vi "Add Data to Table.vi"(10 "User Data":T1(array[cluster])=[{"User ID (key)"=0, "First Name"="Dude", "Last Name"="marlow", "Extension"="", "Department"="", "Citizenship"="", "Company"="", "GDLS Employee"=FALSE, "Foreign National"=FALSE}, {"User ID (key)"=0, "First Name"="Where's", "Last Name"="Nowak", "Extension"="", "Department"="", "Citizenship"="", "Company"="", "GDLS Employee"=FALSE, "Foreign National"=FALSE}, {"User ID (key)"=0, "First Name"="My", "Last Name"="Jones", "Extension"="", "Department"="", "Citizenship"="", "Company"="", "GDLS Employee"=FALSE, "Foreign National"=FALSE}, {"User ID (key)"=0, "First Name"="Car", "Last Name"="Hofer", "Extension"="", "Department"="", "Citizenship"="", "Company"="", "GDLS Employee"=FALSE, "Foreign National"=FALSE}, {"User ID (key)"=0, "First Name"="Man", "Last Name"="Murphy", "Extension"="", "Department"="", "Citizenship"="", "Company"="", "GDLS Employee"=FALSE, "Foreign National"=FALSE}]) -> ()   [LabVIEW 2011]
uses:
  System.Windows.Forms
  System.Data
panel:
  out "CurrentRowIndex":i32
  in  "stop":bool
  in  ".NET Container":refnum<k24>(container)
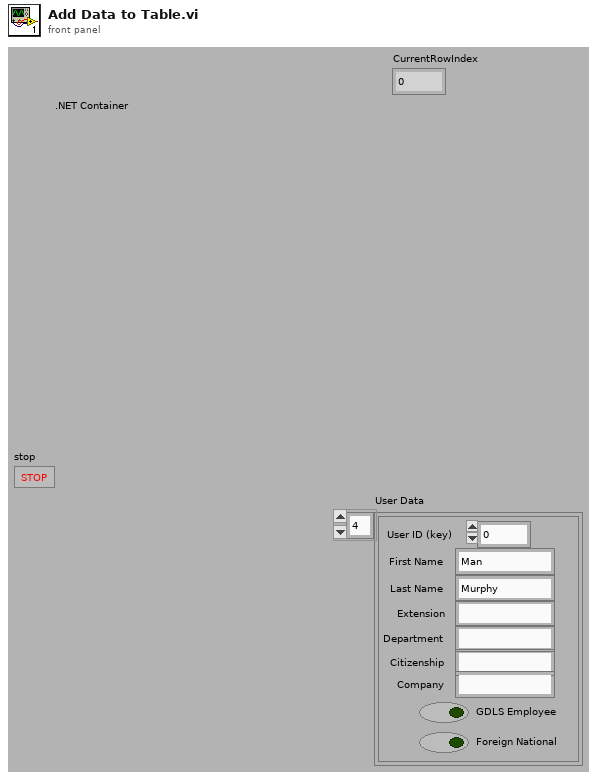
[diagram p1: front panel]
types:
  T1 = cluster{"User ID (key)":i32, "First Name":string, "Last Name":string, "Extension":string, "Department":string, "Citizenship":string, "Company":string, "GDLS Employee":bool, "Foreign National":bool}[]
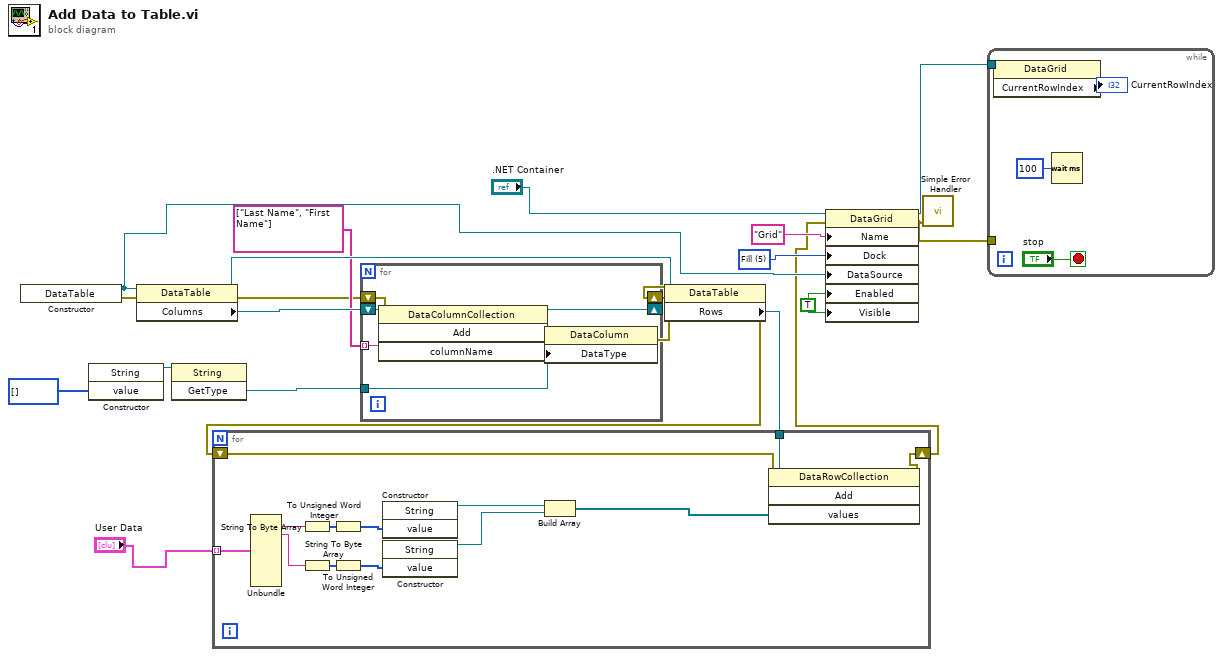
[diagram p0: block diagram]
diagram:
  w9 = TRUE ("Visible")
  w7 = 5 items=["None", "Top", "Bottom", "Left", "Right", "Fill"] ("Dock")
  n1 = constructor class="DataTable"() -> (reference out=w6:refnum<k24>, error out=w5:errorcluster)  [unwired: 3 in, 1 out]
  n2 = constructor class="String"("value"=u16[] [] ("Char[] value")) -> (reference out=w15:refnum<k24>)  [unwired: 3 in, 3 out]
  n3 = property class="DataTable"(reference=w6, error in=w5) -> (reference out=w18:refnum<k24>, error out=w13:errorcluster, "Columns"=w20:refnum<k24>)
  n4 = invoke class="String" method="GetType"(reference=w15) -> ("GetType"=w19:refnum<k24>)  [unwired: 2 in, 2 out]
  n5 = for {
    tunnel: w19 -> [w26]
    tunnel: string[] ["Last Name", "First Name"] -> [w25] mode=indexing
    shift-right: [w21] -> _
    shift-left: w20 -> [w28]
    shift-right: [w22] -> w12
    shift-left: w13 -> [w24]
    n6 = invoke class="DataColumnCollection" method="Add"(reference=w28, error in=w24, "columnName"=w25) -> (reference out=w21:refnum<k24>, error out=w23:errorcluster, "Add"=w27:refnum<k24>)  [unwired: 1 in, 1 out]
    n7 = property class="DataColumn"(reference=w27, error in=w23, "DataType"=w26) -> (error out=w22:errorcluster)  [unwired: 1 out]
  }
  n8 = property class="DataTable"(reference=w18, error in=w12) -> (error out=w4:errorcluster, "Rows"=w17:refnum<k24>)  [unwired: 1 out]
  n9 = for {
    tunnel: w17 -> [w41]
    tunnel: "User Data" -> [w29] mode=indexing
    shift-right: [w31] -> w1
    shift-left: w4 -> [w30]
    n10 = Unbundle(w29) -> ("First Name"=w40:string, "Last Name"=w33:string)  [unwired: 7 out]
    n11 = String To Byte Array(string=w40) -> (unsigned byte array=w39:u8[])
    n12 = String To Byte Array(string=w33) -> (unsigned byte array=w34:u8[])
    n13 = To Unsigned Word Integer(number=w39) -> (unsigned 16bit integer=w38:u16[])
    n14 = To Unsigned Word Integer(number=w34) -> (unsigned 16bit integer=w35:u16[])
    n15 = constructor class="String"("value"=w38) -> (reference out=w37:refnum<k24>)  [unwired: 3 in, 3 out]
    n16 = constructor class="String"("value"=w35) -> (reference out=w32:refnum<k24>)  [unwired: 3 in, 3 out]
    n17 = Build Array(w37, w32) -> (w36:refnum<k24>[])
    n18 = invoke class="DataRowCollection" method="Add"(reference=w41, error in=w30, "values"=w36) -> (error out=w31:errorcluster)  [unwired: 1 in, 3 out]
  }
  n19 = property class="DataGrid"(reference=".NET Container", error in=w1, "Name"="Grid", "Dock"=w7, "DataSource"=w6, "Enabled"=w9, "Visible"=w9) -> (reference out=w3:refnum<k24>, error out=w10:errorcluster)
  n20 = call <vilib>:"Simple Error Handler.vi"("error in (no error)"=w10) -> ()  [unwired: 4 in, 5 out]
  n21 = while {
    tunnel: w10 -> [_]
    tunnel: w3 -> [w42]
    stop <- "stop" stop-if-true
    n22 = property class="DataGrid"(reference=w42) -> ("CurrentRowIndex"=→"CurrentRowIndex":i32)  [unwired: 1 in, 2 out]
    n23 = Wait (ms)(milliseconds to wait=u32 100) -> ()  [unwired: 1 out]
  }
